vi "Wait Cmd Exe.vi"(8 "error in (no error)":errorcluster, 11 "VISA resource name":refnum<visa-resource-name>) -> (0 "error out":errorcluster, 3 "VISA resource name out":refnum<visa-resource-name>, 4 "Device Errors":cluster{"code":i32, "Text":string}[](array[cluster]))   [LabVIEW 2014, in "Stanford Research DG645 - Driver.lvlib"]
doc: "Common IEEE-488.2 Command: *WAI\nInstrument Error Check\n\nThe instrument will not process further commands until all prior commands including this one have completed."
uses:
  Stanford Research DG645 - Driver.lvlib
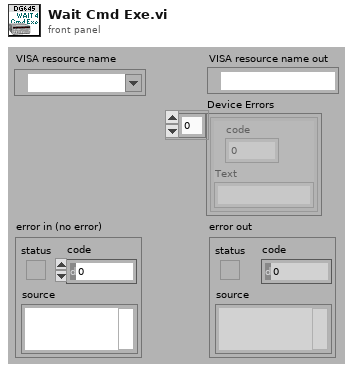
[diagram p1: front panel]
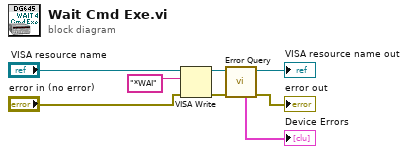
[diagram p0: block diagram]
diagram:
  n1 = VISA Write(VISA resource name="VISA resource name", write buffer="*WAI" ("command"), error in (no error)="error in (no error)") -> (VISA resource name out=w6:refnum<visa-resource-name>, error out=w3:errorcluster)  [unwired: 1 out]
  n2 = call "Error Query.vi"("error in (no error)"=w3, "VISA resource name"=w6) -> ("error out"=→"error out":errorcluster, "VISA resource name out"=→"VISA resource name out":refnum<visa-resource-name>, "Device Errors"=→"Device Errors":cluster{"code":i32, "Text":string}[])  [unwired: 7 in]
